vi "solar Voyager Launch.vi"(8 "error in (no error)":errorcluster, 11 "solar in":refnum<class "solar.lvclass">) -> (0 "error out":errorcluster, 3 "solar out":refnum<class "solar.lvclass">)   [LabVIEW 2018]
doc: "This launches the Voyager interface. If the Voyager key is not found in the configuration file, the default configuration is a single TCP Server on port 59200 for each target. Voyager has four configurations:\n- SERVER - TCP server that handles commands and telemetry\n- CLIENT - TCP client that handles commands and telemetry (IP address required)\n- SERVER_CMD - TCP server that only handles incoming commands\n- SERVER_TLM - TCP server that only handles outgoing telemetry"
uses:
  voyager/solar_voy_ctl Port.ctl
  voyager/solar_voy_ctl Port Setup.ctl
  cfg/solar_cfg Read File (Str).vi
  solar.lvclass
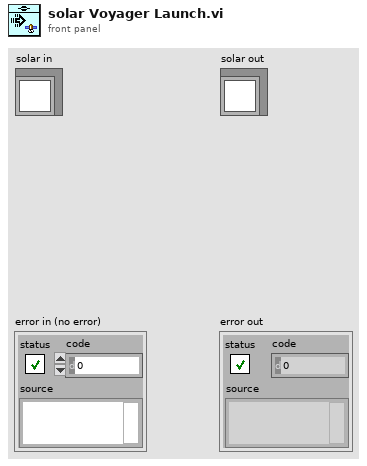
[diagram p1: front panel]
types:
  T1 = typedef "solar_voy_ctl Voyager Refnum.ctl" = refnum<k1>
  T2 = typedef "solar_voy_ctl Port Setup.ctl" = enum8{"SERVER", "CLIENT", "SERVER_CMD", "SERVER_TLM"}
  T3 = typedef "solar_voy_ctl Port.ctl" = cluster{"Setup":T2, "Port":u16, "ServerIP":string, "Target":string}
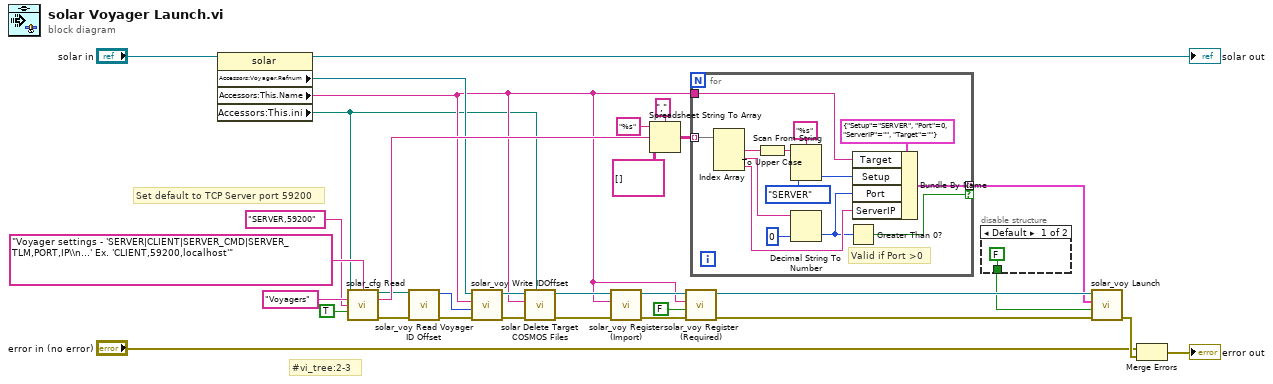
[diagram p0: block diagram]
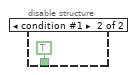
[diagram p2: hidden frame]
diagram:
  # "#vi_tree:2-3"
  # "Set default to TCP Server port 59200"
  n1 = property class="solar"(reference="solar in") -> (reference out=→"solar out":refnum<class "solar.lvclass">, "Accessors:Voyager.Refnum"=w8:T1, "Accessors:This.Name"=w3:string, "Accessors:This.ini"=w2:path)  [unwired: 1 in, 1 out]
  n2 = call-poly "solar_cfg Read.vi"("Config Path (*.ini)"=w2, "Comment"="Voyager settings - 'SERVER|CLIENT|SERVER_CMD|SERVER_TLM,PORT,IP\\n...' Ex. 'CLIENT,59200,localhost'", "Key"="Voyagers", "Value in"="SERVER,59200", "Add Quotes? (T)"=TRUE) -> ("Config Path out"=w12:path, "Value out"=w17:string, "error out"=w11:errorcluster)  [unwired: 7 in, 1 out]
  n3 = call "solar_voy Read Voyager ID Offset.vi"("error in (no error)"=w11, "Config Path in"=w12) -> ("error out"=w10:errorcluster, "VoyagerIDOffset"=w9:u16)  [unwired: 8 in]
  n4 = call "solar_voy Write IDOffset.vi"("error in (no error)"=w10, "ID Offset"=w9, "Target Name"=w3, "Voyager Refnum in"=w8) -> ("error out"=w7:errorcluster, "Voyager Refnum out"=w5:T1)  [unwired: 6 in]
  n5 = call "solar Delete Target COSMOS Files.vi"("Config Path"=w2, "error in (no error)"=w7, "Target"=w3, "Refnum in"=w5) -> ("error out"=w6:errorcluster, "Refnum out"=w4:T1)  [unwired: 6 in]
  n6 = call "solar_voy Register (Import).vi"("error in (no error)"=w6, "Target Name"=w3, "Voyager Refnum in"=w4) -> ("error out"=w29:errorcluster, "Voyager Refnum out"=w28:T1)  [unwired: 7 in]
  n7 = Spreadsheet String To Array(delimiter (Tab)=",", format string="%s", spreadsheet string=w17, array type (2D Dbl)=string[][] []) -> (array=w21:string[][])
  n8 = call "solar_voy Register (Required).vi"("error in (no error)"=w29, "Override If Exists? (F)"=FALSE, "Target Name"=w3, "Voyager Refnum in"=w28) -> ("error out"=w27:errorcluster, "Voyager Refnum out"=w26:T1)  [unwired: 6 in]
  n9 = for {
    tunnel: w21 -> [w46] mode=indexing
    tunnel: [w40] -> w15 mode=indexing if=w39
    tunnel: w3 -> [w33]
    # "Valid if Port >0"
    n10 = Index Array(array=w46) -> (element #1=w38:string, element #2=w45:string, element #3=w42:string)  [unwired: 3 in]
    n11 = To Upper Case(1:w38) -> (0:w36:string)
    n12 = Scan From String(format string="%s", input string=w36, default 1=solar_voy_ctl_Port_Setup."SERVER" ("Setup")) -> (output 1=w34:T2)  [unwired: 2 in, 3 out]
    n13 = Decimal String To Number(string=w45, default (0L)=u16 0 ("Port")) -> (number=w41:u16)  [unwired: 1 in, 1 out]
    n14 = Greater Than 0?(x=w41) -> (x > 0?=w39:bool)
    n15 = Bundle By Name(cluster=T3 {"Setup"=enum."SERVER", "Port"=0, "ServerIP"="", "Target"=""} ("Port"), "Target"=w33, "Setup"=w34, "Port"=w41, "ServerIP"=w42) -> (w40:T3)
  }
  n16 = disable-structure shown="Default" {
    disable-tunnel: [FALSE TRUE ("Open FP? (F)")] -> w13
    frame condition #0 (active) {
    }
    frame condition #1 {
    }
  }
  n17 = call "solar_voy Launch.vi"("error in (no error)"=w27, "Open FP? (F)"=w13, "Ports"=w15, "Voyager Refnum in"=w26) -> ("error out"=w30:errorcluster)  [unwired: 6 in, 1 out]
  n18 = Merge Errors("error in (no error)", w30) -> (→"error out":errorcluster)
